vi "Get Data Out from Voltage and V Ref.vi"(10 "Vref (V)":dbl, 11 "Voltage (V)":dbl) -> (3 "Data Out (14-bit)":u16)   [LabVIEW 2017, in "Host SRL.lvlib"]
uses:
  Host SRL.lvlib
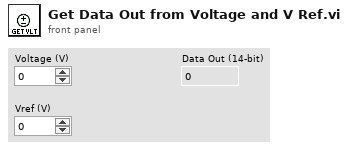
[diagram p1: front panel]
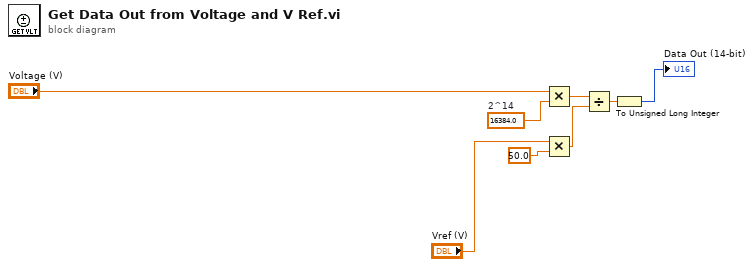
[diagram p0: block diagram]
diagram:
  w1 = 16384.0  # 2^14
  n1 = Multiply(x="Voltage (V)", y=w1) -> (x*y=w4:dbl)
  n2 = Multiply(x="Vref (V)", y=50.0 ("x")) -> (x*y=w3:dbl)
  n3 = Divide(x=w4, y=w3) -> (x/y=w5:dbl)
  n4 = To Unsigned Long Integer(number=w5) -> (unsigned 32bit integer=→"Data Out (14-bit)":u32)
